vi "Compute I path (SubVI).vi"(9 "I step":dbl=1.0, 10 "wpt":refnum<queue>, 11 "Path":refnum<queue>) -> ()   [LabVIEW 2011]
uses:
  Trap cluster.ctl
panel:
  out "Numeric":i32
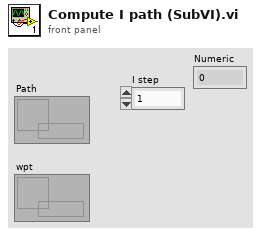
[diagram p1: front panel]
types:
  T1 = typedef "Trap cluster.ctl" = cluster{"X (IMAQ)":sgl[], "Y (IMAQ)":sgl[], "Z":sgl[], "I":sgl[], "Trap number":i32[], "ROI number":i32[], "Number of traps":i32, "Group":bool[]}
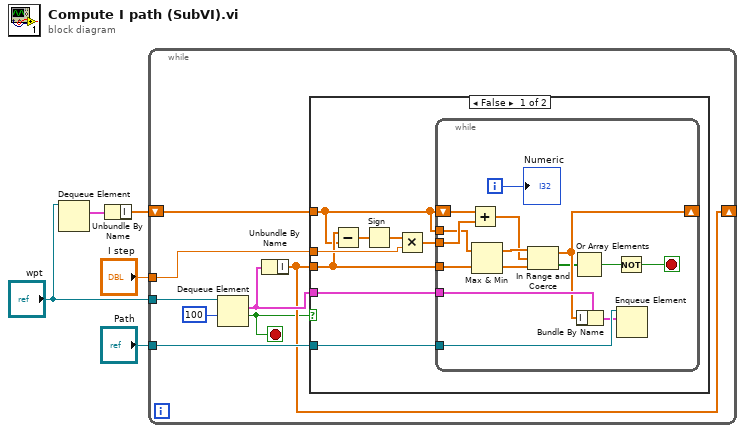
[diagram p0: block diagram]
diagram:
  n1 = Dequeue Element(queue="wpt") -> (element=w4:T1)  [unwired: 2 in, 3 out]
  n2 = Unbundle By Name(w4) -> ("I"=w3:sgl[])
  n3 = while {
    tunnel: "wpt" -> [w13]
    tunnel: "I step" -> [w11]
    tunnel: "Path" -> [w9]
    shift-right: [w7] -> _
    shift-left: w3 -> [w10]
    stop <- w6 stop-if-true
    n4 = Dequeue Element(queue=w13, timeout in ms (-1)=100) -> (element=w8:T1, timed out?=w6:bool)  [unwired: 1 in, 2 out]
    n5 = Unbundle By Name(w8) -> ("I"=w7:sgl[])
    n6 = case shown="False" w6 {
      tunnel: w11 -> [w19 _]
      tunnel: w10 -> [w14 _]
      tunnel: w9 -> [w17 _]
      tunnel: w8 -> [w16 _]
      tunnel: w7 -> [w15 _]
      frame False {
        n7 = Subtract(x=w15, y=w14) -> (x-y=w20:sgl[])
        n8 = Sign(1:w20) -> (0:w21:sgl[])
        n9 = Multiply(x=w21, y=w19) -> (x*y=w18:dbl[])
        n10 = while {
          tunnel: w18 -> [w36]
          tunnel: w14 -> [w24]
          tunnel: w17 -> [w31]
          tunnel: w16 -> [w29]
          shift-right: [w28] -> _
          shift-left: w14 -> [w25]
          tunnel: w15 -> [w22]
          i -> [w23]
          stop <- w26 stop-if-true
          n11 = Add(x=w25, y=w36) -> (x+y=w33:dbl[])
          n12 = Max & Min(x=w24, y=w22) -> (max(x,y)=w35:sgl[], min(x,y)=w34:sgl[])
          n13 = In Range and Coerce(upper limit=w35, x=w33, lower limit=w34) -> (coerced(x)=w28:dbl[], In Range?=w27:bool[])
          n14 = Or Array Elements(Boolean array=w27) -> (logical OR=w32:bool)
          n15 = Bundle By Name(cluster=w29, "I"=w28) -> (w30:T1)
          n16 = Not(x=w32) -> (.not. x?=w26:bool)
          n17 = Enqueue Element(queue=w31, element=w30) -> ()  [unwired: 2 in, 3 out]
          "Numeric" <- w23
        }
      }
      frame True {
      }
    }
  }
